vi "Remove All Channels.vi"(8 "error in (no error)":errorcluster, 11 "Item Ref in":T1 format="%.0x") -> (0 "error out":errorcluster, 3 "Item Ref out":T1 format="%.0x")   [LabVIEW 2027, in "System Monitor System Explorer.lvlib"]
uses:
  System Monitor System Explorer.lvlib
  <vilib>/NI VeriStand/Custom Device API/Custom Device Item Ref.ctl
  <vilib>/NI VeriStand/Custom Device API/Custom Device API.lvlib
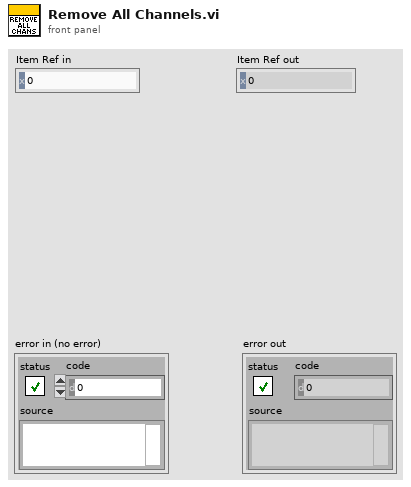
[diagram p1: front panel]
types:
  T1 = typedef "Custom Device API.lvlib/Custom Device Item Ref.ctl" = u64
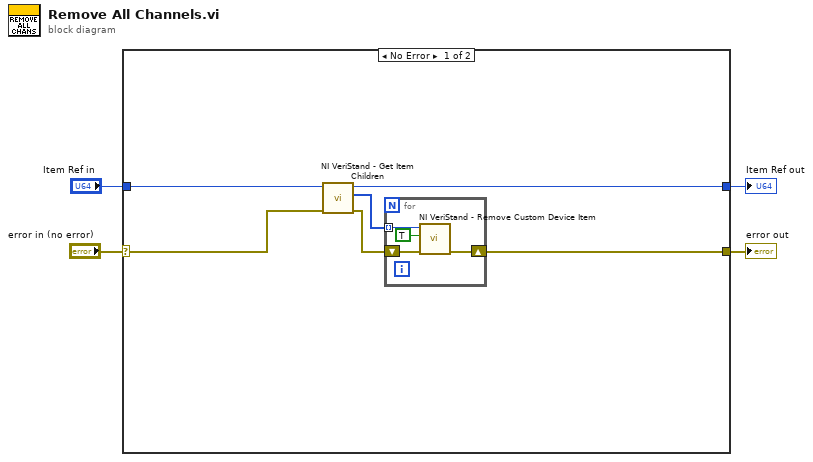
[diagram p0: block diagram]
diagram:
  n1 = case shown="No Error" "error in (no error)" {
    selector: "error in (no error)" -> [w6 w16]
    tunnel: [w5 w16] -> w4
    tunnel: [w9 w15] -> w2
    tunnel: "Item Ref in" -> [w10 w15]
    frame No Error {
      n2 = call <vilib>:"NI VeriStand - Get Item Children.vi"("error in (no error)"=w6, "Item Ref in"=w10) -> ("error out"=w7:errorcluster, "Child Refs"=w8:T1[], "Item Ref out"=w9:T1)  [unwired: 6 in, 1 out]
      n3 = for {
        tunnel: w8 -> [w14] mode=indexing
        shift-right: [w11] -> w5
        shift-left: w7 -> [w12]
        n4 = call <vilib>:"NI VeriStand - Remove Custom Device Item.vi"("error in (no error)"=w12, "Force Delete (F)"=TRUE, "Item Ref in"=w14) -> ("error out"=w11:errorcluster)  [unwired: 7 in, 1 out]
      }
    }
    frame Error {
    }
  }
  "error out" <- w4
  "Item Ref out" <- w2
